vi "Get Sequences.vi"(8 "error in (no error)":errorcluster, 11 "VISA resource name":refnum<visa-resource-name>) -> (0 "error out":errorcluster, 3 "VISA resource name out":refnum<visa-resource-name>, 4 "Byte 3 Delay":u8[](array[numeric]), 5 "Byte 2 Ch.":u8[](array[numeric]), 7 "Byte 1 Ch.":u8[](array[numeric]))   [LabVIEW 2020, in "QuPMXdriver.lvlib"]
doc: "Gets all sequences from multiplexer and return bytes."
uses:
  QuPMXdriver.lvlib
  <vilib>/Utility/error.llb/Error Cluster From Error Code.vi
  <vilib>/ErrorRing/Error Ring.xnode
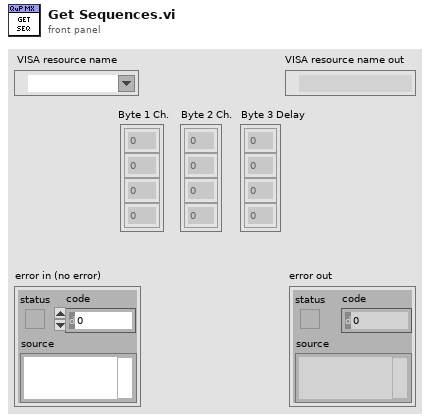
[diagram p1: front panel]
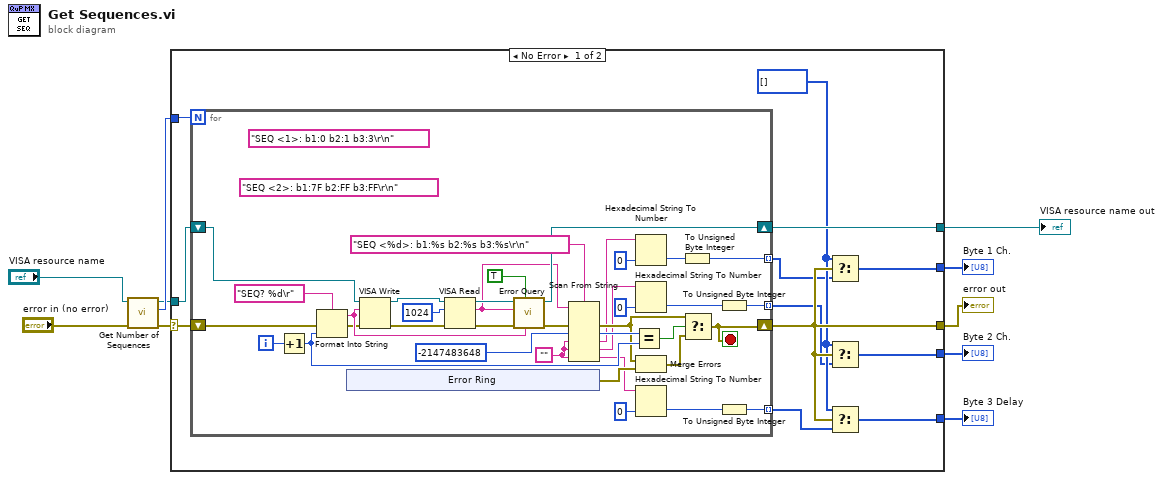
[diagram p0: block diagram]
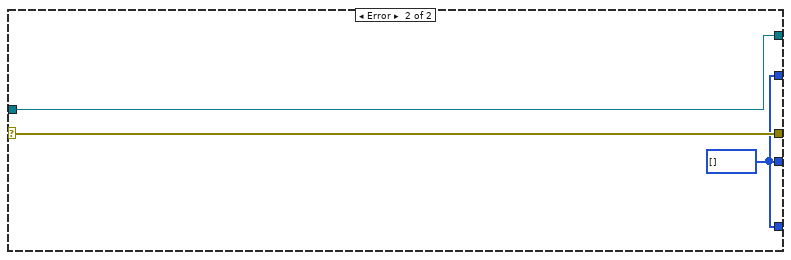
[diagram p2: hidden frame]
diagram:
  n1 = call "Get Number of Sequences.vi"("error in (no error)"="error in (no error)", "VISA resource name"="VISA resource name") -> ("error out"=w8:errorcluster, "Number of sequences"=w7:i32, "VISA resource name out"=w6:refnum<visa-resource-name>)  [unwired: 7 in]
  n2 = case shown="No Error" w8 {
    selector: w8 -> [w21 w67]
    tunnel: w7 -> [w22 _]
    tunnel: w6 -> [w20 w66]
    tunnel: [w19 w66] -> w5
    tunnel: [w18 w67] -> w4
    tunnel: [w15 w65] -> w3
    tunnel: [w16 w65] -> w2
    tunnel: [w17 w65] -> w1
    frame No Error {
      w14 = u8[] [] ("f")
      n3 = for {
        N: w22 -> [_]
        shift-right: [w39] -> w18
        shift-left: w21 -> [w50]
        shift-right: [w47] -> w19
        shift-left: w20 -> [w48]
        tunnel: [w38] -> w13 mode=indexing
        tunnel: [w37] -> w12 mode=indexing
        tunnel: [w36] -> w11 mode=indexing
        i -> [w53]
        stop <- w39 stop-if-true
        w27 = ""
        (unwired) "SEQ <2>: b1:7F b2:FF b3:FF\r\n"
        (unwired) "SEQ <1>: b1:0 b2:1 b3:3\r\n"
        n4 = Increment(x=w53) -> (x+1=w44:i32)
        n5 = Format Into String(format string="SEQ? %d\r", error in=w50, w44) -> (resulting string=w51:string, error out=w49:errorcluster)  [unwired: 1 in]
        n6 = xnode "Error Ring"() -> ("error out"=w42:errorcluster)
        n7 = VISA Write(VISA resource name=w48, write buffer=w51, error in (no error)=w49) -> (VISA resource name out=w58:refnum<visa-resource-name>, error out=w54:errorcluster)  [unwired: 1 out]
        n8 = VISA Read(VISA resource name=w58, byte count=u32 1024, error in (no error)=w54) -> (VISA resource name out=w57:refnum<visa-resource-name>, read buffer=w34:string, error out=w56:errorcluster)  [unwired: 1 out]
        n9 = call "Error Query.vi"("Last command"=w51, "Ignore empty sequence? (T)"=TRUE, "error in (no error)"=w56, "Read buffer"=w34, "VISA resource name"=w57) -> ("error out"=w46:errorcluster, "VISA resource name out"=w47:refnum<visa-resource-name>)  [unwired: 5 in]
        n10 = Scan From String(format string="SEQ <%d>: b1:%s b2:%s b3:%s\r\n", input string=w34, error in=w46, default 1=-2147483648 ("default value 1"), default 2=w27, default 3=w27, default 4=w27) -> (error out=w41:errorcluster, output 1=w45:i32, output 2=w33:string, output 3=w31:string, output 4=w29:string)  [unwired: 1 in, 2 out]
        n11 = Equal?(x=w45, y=w44) -> (x = y?=w43:bool)
        n12 = Hexadecimal String To Number(string=w33, default (0uL)=u32 0 ("default (0 U32)")) -> (number=w32:u32)  [unwired: 1 in, 1 out]
        n13 = Hexadecimal String To Number(string=w31, default (0uL)=u32 0 ("default (0 U32)")) -> (number=w30:u32)  [unwired: 1 in, 1 out]
        n14 = Merge Errors(w41, w42) -> (w40:errorcluster)
        n15 = Hexadecimal String To Number(string=w29, default (0uL)=u32 0 ("default (0 U32)")) -> (number=w28:u32)  [unwired: 1 in, 1 out]
        n16 = To Unsigned Byte Integer(number=w32) -> (unsigned 8bit integer=w38:u8)
        n17 = Select(t=w41, s=w43, f=w40) -> (s? t:f=w39:errorcluster)
        n18 = To Unsigned Byte Integer(number=w30) -> (unsigned 8bit integer=w37:u8)
        n19 = To Unsigned Byte Integer(number=w28) -> (unsigned 8bit integer=w36:u8)
      }
      n20 = Select(t=w14, s=w18, f=w13) -> (s? t:f=w15:u8[])
      n21 = Select(t=w14, s=w18, f=w12) -> (s? t:f=w16:u8[])
      n22 = Select(t=w14, s=w18, f=w11) -> (s? t:f=w17:u8[])
    }
    frame Error {
      w65 = u8[] []
    }
  }
  "error out" <- w4
  "VISA resource name out" <- w5
  "Byte 1 Ch." <- w3
  "Byte 2 Ch." <- w2
  "Byte 3 Delay" <- w1
